vi "DMM Acq Done_old_2_5_2021.vi"(9 "Acquisition State":T1, 10 "Backlog":i32, 11 "Channel Index":i32) -> (2 "Finished with Backlog?":bool, 3 "Sequence Acquision Finished?":bool)   [LabVIEW 2019, in "SupportVIs.lvlib"]
uses:
  SupportVIs.lvlib
  <instrlib>/niDMM/nidmm.llb/niDMM Acquisition State.ctl
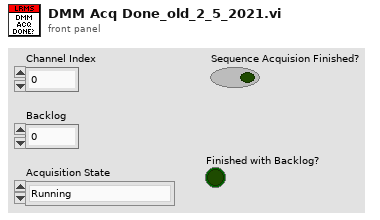
[diagram p1: front panel]
types:
  T1 = typedef "niDMM Acquisition State.ctl" = enum16{"Running", "Finished with Backlog", "Finished with no Backlog", "Paused", "No acquisition in progress"}
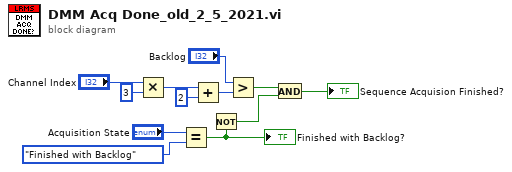
[diagram p0: block diagram]
diagram:
  n1 = Multiply(x="Channel Index", y=3) -> (x*y=w8:i32)
  n2 = Equal?(x="Acquisition State", y=niDMM_Acquisition_State."Finished with Backlog") -> (x = y?=w1:bool)
  "Finished with Backlog?" <- w1
  n3 = Add(x=w8, y=2) -> (x+y=w7:i32)
  n4 = Not(x=w1) -> (.not. x?=w2:bool)
  n5 = Greater?(x="Backlog", y=w7) -> (0:w11:bool)
  n6 = And(x=w11, y=w2) -> (x .and. y?=→"Sequence Acquision Finished?":bool)
